vi "basic - Transmit.vi"() -> ()   [LabVIEW 2020]
uses:
  src/_polimorphicInstances/control/Fdx Start (Tx).vi
  src/AIM664LV.lvlib
  src/_polimorphicInstances/session/Fdx Create Session (Tx-Generic).vi
  src/_polimorphicInstances/session/Fdx Close Session (Port).vi
  src/_polimorphicInstances/control/Fdx Stop (Tx).vi
  src/_controls/queue_data_full.ctl
  src/_controls/queue_header_generic.ctl
panel:
  out "Transmitted Frame":string[][](table)
  out "Frame":u8[](array[numeric]) format="%.0x"
  in  "PortMap":u32
  out "Duplicated":bool
  in  "size":i32=100
  in  "HeaderInfo":T1={"InterFrameGap"=25, "PacketGroupWaitTime"=5000, "PayloadBufferMode"=0, "PayloadGenerationMode"=0, "PreambleCount"=7, "Skew"=0, "NetSelect"=3, "FrameStartMode"=1, "PhysErrorInjection"=0, "SequenceNumberInit"=65535, "SequenceNumberOffset"=65535} {"NetSelect" items=["FDX_TX_FRAME_DLY_A"=0, "FDX_TX_FRAME_DLY_B"=1, "FDX_TX_FRAME_BOTH "=3, "FDX_TX_FRAME_ONLY_A"=4, "FDX_TX_FRAME_ONLY_B "=5]; "FrameStartMode" items=["FDX_TX_FRAME_START_IFG", "FDX_TX_FRAME_START_PGWT", "FDX_TX_FRAME_START_TRG"]; "PhysErrorInjection" items=["FDX_TX_FRAME_ERR_OFF"=0, "FDX_TX_FRAME_ERR_CRC"=1, "FDX_TX_FRAME_ERR_ALI"=2, "FDX_TX_FRAME_ERR_PRE"=4, "FDX_TX_FRAME_ERR_PHY"=8]; "SequenceNumberInit" items=["FDX_TX_FRAME_SEQ_INIT_AUTO"=65535]; "SequenceNumberOffset" items=["FDX_TX_FRAME_SEQ_OFFS_AUTO "=65535]; "PayloadGenerationMode" items=["FDX_TX_FRAME_PGM_USER"=0, "FDX_TX_FRAME_PGM_IP_PART"=1, "FDX_TX_FRAME_PGM_IP_FULL"=2, "FDX_TX_FRAME_PGM_IP_PART_TT"=10, "FDX_TX_FRAME_PGM_IP_FULL_TT"=20]; "PayloadBufferMode" items=["FDX_TX_FRAME_PBM_STD", "FDX_TX_FRAME_PBM_MAC", "FDX_TX_FRAME_PBM_UDP"]}
  in  "VL Id":u16=60
  in  "Configuration":T2={"domainID"=1, "sideID"=1, "locationID"=1, "interfaceID"=1, "partitionID"=1} {"interfaceID" format="%.0b"}
  out "Payload":u8[](array[numeric]) format="%.0x"
  in  "UDPdstPort":u16=1
  in  "UDPsrcPort":u16=1
  out "TxStatus":T3={"TxStatus"=1, "Frames"=855, "TransmitMode"=0, "FramesPortB"=0}
  out "TxQueueStatus":T4={"QueueStatus"=0, "BytesReloadable"=0, "FramesSent"=854, "FramesInCycQueue"=0} {"QueueStatus" items=["FDX_QUE_EMPTY", "FDX_QUE_FILLED", "FDX_QUE_FULL", "FDX_QUE_SENT", "FDX_QUE_CYCL_RUN", "FDX_QUE_CYCL_SENT"]}
  out "TxQueueInfo":cluster{"QueueBaseAddr":u32, "QueueSizeOut":u32}={"QueueBaseAddr"=50892800, "QueueSizeOut"=4194304}
  out "QueueSizeIn":u32
  in  "Port":u32
  in  "Board":u32
  out "current time":timestamp=timestamp(3686777794.875688 s since 1904-01-01)
  out "current irig time":T5={"SignOut"=40, "DayOut"=1, "HourOut"=1, "MinOut"=28, "SecondOut"=39, "MilliSecOut"=539, "MicroSecOut"=300, "NanoSecOut"=0, "InfoOut"=0, "Mode"=3}
  in  "stop":bool
  out "PortInitOut":T6={"PortConfig"=0, "PortUsed"=1, "GlobalMemFree"=0, "SharedMemFree"=0} {"PortConfig" items=["FDX_SINGLE", "FDX_REDUNDANT"]}
  out "error out":errorcluster
  # "ARINC 664 - Transmitting Frames"
  # "Overview: Setup the board to transmit package as raw frames.\nRequirement: One AIM ARINC-664 board with installed AIM ARINC 664 BSP.\nRestrictions: None.\nInstruction:\n1. Select the Board ID (0 if you have only one board in your system) and the port number. If you want to validate between two ports in one device, you can use tx board and Rx Board\n2. Run the VI.\n3. See the result in Current IRIG Time"
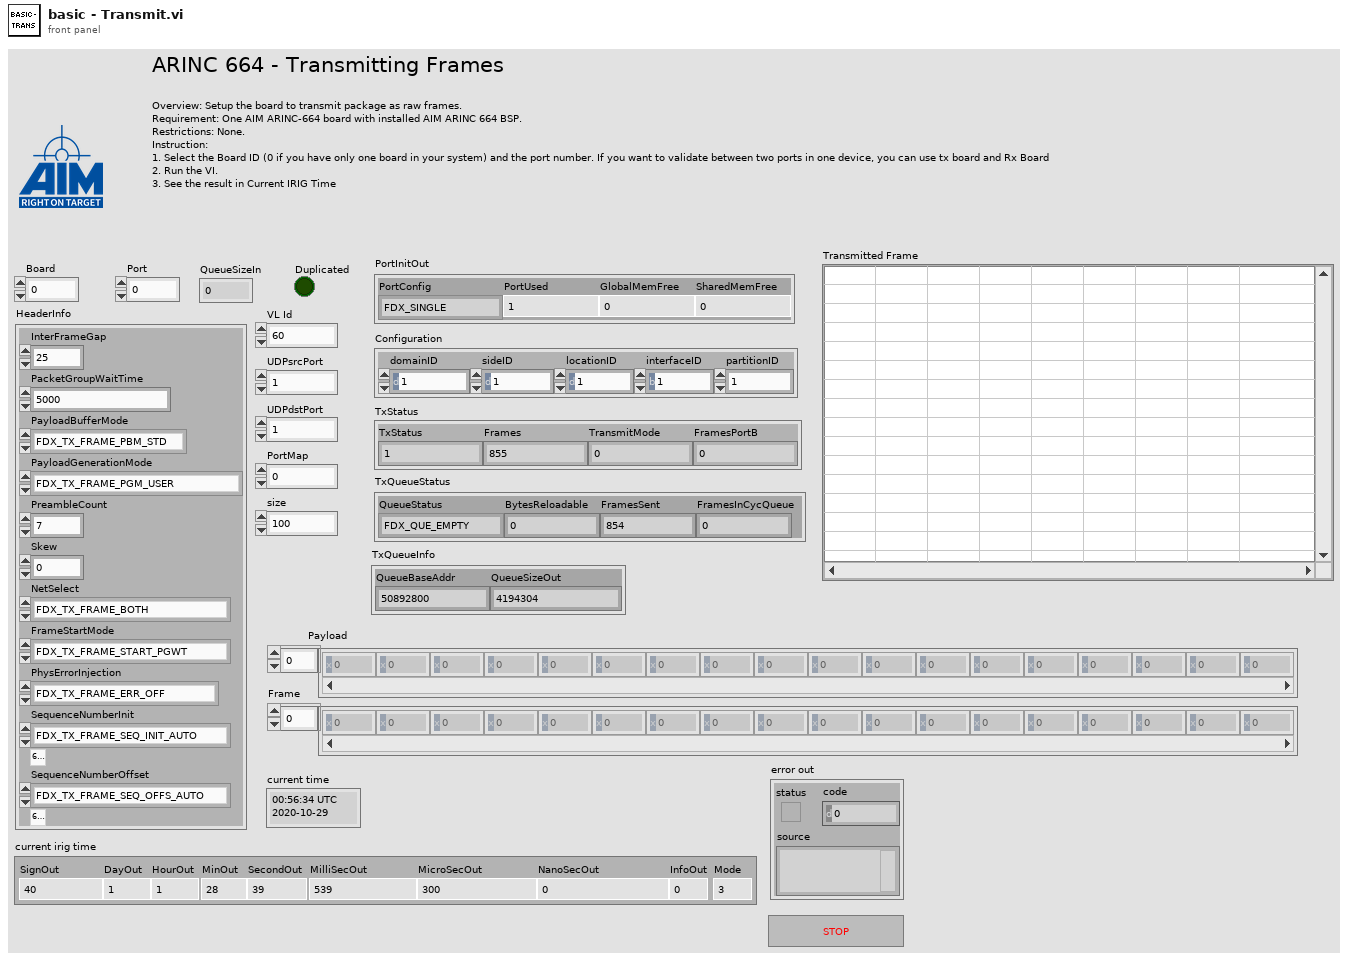
[diagram p1: front panel]
types:
  T1 = typedef "AIM664LV.lvlib/queue_header_generic.ctl" = cluster{"InterFrameGap":u32, "PacketGroupWaitTime":u32, "PayloadBufferMode":u8, "PayloadGenerationMode":u8, "PreambleCount":u8, "Skew":u32, "NetSelect":u8, "FrameStartMode":u8, "PhysErrorInjection":u32, "SequenceNumberInit":u16, "SequenceNumberOffset":u16}
  T2 = typedef "AIM664LV.lvlib/queue_data_full.ctl" = cluster{"domainID":u8, "sideID":u8, "locationID":u8, "interfaceID":u8, "partitionID":u8}
  T3 = cluster{"TxStatus":u32, "Frames":u32, "TransmitMode":u32, "FramesPortB":u32}
  T4 = cluster{"QueueStatus":i32, "BytesReloadable":u32, "FramesSent":u32, "FramesInCycQueue":u32}
  T5 = cluster{"SignOut":i32, "DayOut":u32, "HourOut":u32, "MinOut":u32, "SecondOut":u32, "MilliSecOut":u32, "MicroSecOut":u32, "NanoSecOut":u32, "InfoOut":u32, "Mode":u32}
  T6 = cluster{"PortConfig":u32, "PortUsed":u32, "GlobalMemFree":u32, "SharedMemFree":u32}
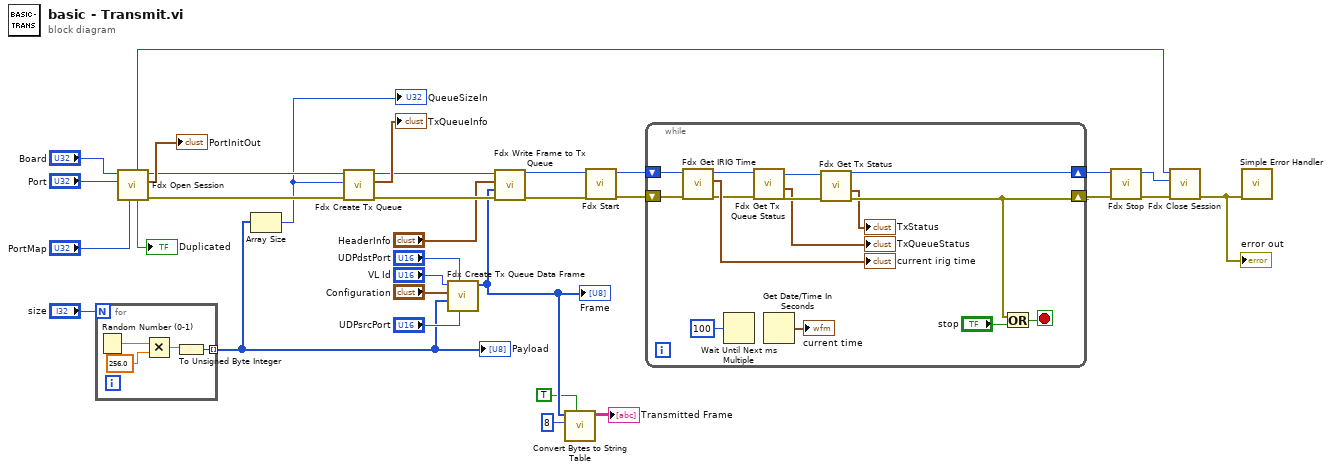
[diagram p0: block diagram]
diagram:
  n1 = for {
    N: "size" -> [_]
    tunnel: [w33] -> w11 mode=indexing
    n2 = Random Number (0-1)() -> (number: 0 to 1=w36:dbl)
    n3 = Multiply(x=w36, y=256.0) -> (x*y=w34:dbl)
    n4 = To Unsigned Byte Integer(number=w34) -> (unsigned 8bit integer=w33:u8)
  }
  "Payload" <- w11
  n5 = call-poly "Fdx Open Session.vi"("PortMap"="PortMap", "port"="Port", "board"="Board") -> ("error out"=w26:errorcluster, "PortInitOut"=→"PortInitOut":T6, "port handle out"=w27:u32, "Duplicated"=→"Duplicated":bool, "InstrumentHandle_board out"=w6:u32)  [unwired: 4 in]
  n6 = Array Size(array=w11) -> (size(s)=w13:i32)
  "QueueSizeIn" <- w13
  n7 = call "Fdx Create Tx Queue.vi"("error in (no error)"=w26, "QueueSizeIn"=w13, "InstrumentHandle_port in"=w27) -> ("error out"=w24:errorcluster, "TxQueueInfo"=→"TxQueueInfo":cluster{"QueueBaseAddr":u32, "QueueSizeOut":u32}, "InstrumentHandle_port out"=w21:u32)  [unwired: 6 in]
  n8 = call "Fdx Create Tx Queue Data Frame.vi"("UDPsrcPort"="UDPsrcPort", "UDPdstPort"="UDPdstPort", "Payload"=w11, "afdx configuration"="Configuration", "VL Id"="VL Id") -> ("Frame"=w2:u8[])  [unwired: 6 in]
  "Frame" <- w2
  n9 = call "Fdx Write Frame to Tx Queue.vi"("error in (no error)"=w24, "Frame in"=w2, "HeaderInfo"="HeaderInfo", "InstrumentHandle_port in"=w21) -> ("error out"=w23:errorcluster, "InstrumentHandle_port out"=w22:u32)  [unwired: 6 in]
  n10 = call "Convert Bytes to String Table.vi"("Append ASCII Column?"=TRUE, "byters per row"=8, "Data"=w2) -> ("Data"=→"Transmitted Frame":string[][])  [unwired: 8 in]
  n11 = call-poly "Fdx Start.vi"("error in (no error)"=w23, "InstrumentHandle_port in"=w22) -> ("error out"=w31:errorcluster, "InstrumentHandle_port out"=w30:u32)  [unwired: 8 in]
  n12 = while {
    shift-right: [w41] -> w19
    shift-left: w30 -> [w37]
    shift-right: [w42] -> w20
    shift-left: w31 -> [w38]
    stop <- w50 stop-if-true
    n13 = call "Fdx Get IRIG Time.vi"("error in (no error)"=w38, "InstrumentHandle_board in"=w37) -> ("error out"=w45:errorcluster, "Curent Irig Time"=→"current irig time":T5, "InstrumentHandle_board out"=w46:u32)  [unwired: 7 in]
    n14 = Wait Until Next ms Multiple(millisecond multiple=u32 100) -> ()  [unwired: 1 out]
    n15 = call "Fdx Get Tx Queue Status.vi"("error in (no error)"=w45, "InstrumentHandle in"=w46) -> ("error out"=w43:errorcluster, "TxQueueStatus"=→"TxQueueStatus":T4, "InstrumentHandle out"=w44:u32)  [unwired: 7 in]
    n16 = Get Date/Time In Seconds() -> (seconds since 1Jan1904=→"current time":timestamp)
    n17 = call "Fdx Get Tx Status.vi"("error in (no error)"=w43, "InstrumentHandle_port in"=w44) -> ("error out"=w42:errorcluster, "TxStatus"=→"TxStatus":T3, "InstrumentHandle_port out"=w41:u32)  [unwired: 7 in]
    n18 = Or(x=w42, y="stop") -> (x .or. y?=w50:bool)
  }
  n19 = call-poly "Fdx Stop.vi"("error in (no error)"=w20, "InstrumentHandle_port in"=w19) -> ("error out"=w28:errorcluster, "InstrumentHandle_port out"=w8:u32)  [unwired: 8 in]
  n20 = call-poly "Fdx Close Session.vi"("error in (no error)"=w28, "InstrumentHandle_port in"=w8, "InstrumentHandle_board in"=w6) -> ("error out"=w5:errorcluster)  [unwired: 8 in]
  "error out" <- w5
  n21 = call <vilib>:"Simple Error Handler.vi"("error in (no error)"=w5) -> ()  [unwired: 4 in, 5 out]
